vi "滤波参数.vi"(7 "滤波次数":u32=5, 11 "x":dbl format="%0.2f") -> (3 "mode":dbl caption="众数" format="%0.2f")   [LabVIEW 2016, in "斯坦道多参数.lvlib"]
uses:
  <vilib>/Analysis/baseanly.llb/Mean (DBL).vi
  <vilib>/Analysis/NI_AALBase.lvlib
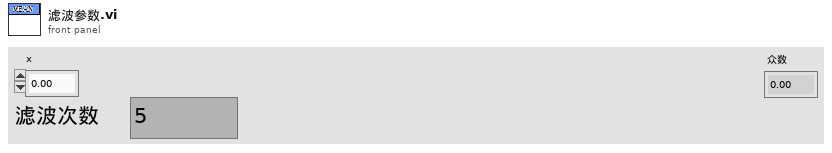
[diagram p1: front panel]
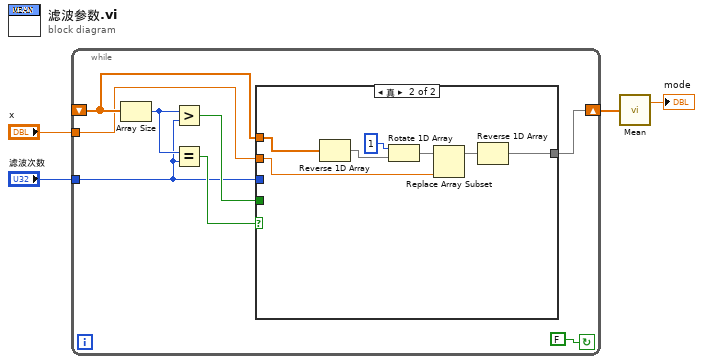
[diagram p0: block diagram]
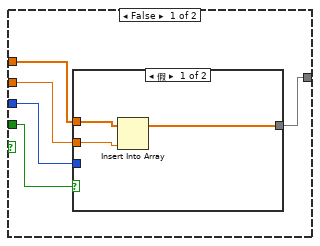
[diagram p2: hidden frame]
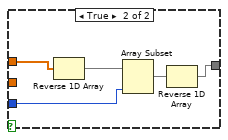
[diagram p3: hidden frame]
diagram:
  n1 = while {
    tunnel: "滤波次数" -> [w5]
    tunnel: "x" -> [w9]
    shift-right: [w8] -> w2
    shift-left: _ -> [w10]
    stop <- FALSE continue-if-true
    n2 = Array Size(array=w10) -> (size(s)=w7:i32)
    n3 = Greater?(x=w7, y=w5) -> (0:w6:bool)
    n4 = Equal?(x=w7, y=w5) -> (x = y?=w11:bool)
    n5 = case shown="真" w11 {
      tunnel: w10 -> [w17 w32]
      tunnel: w9 -> [w16 w30]
      tunnel: [w15 w26] -> w8
      tunnel: w6 -> [w14 _]
      tunnel: w5 -> [w13 _]
      frame False {
        n6 = case shown="假" w14 {
          tunnel: w17 -> [w20 w25]
          tunnel: w16 -> [w19 _]
          tunnel: [w18 w21] -> w15
          tunnel: w13 -> [_ w23]
          frame False {
            n7 = Insert Into Array(array=w20, new element=w19) -> (w18:dbl[])  [unwired: 1 in]
          }
          frame True {
            n8 = Reverse 1D Array(array=w25) -> (reversed array=w24:dbl[])
            n9 = Array Subset(array=w24, length=w23) -> (w22:dbl[])  [unwired: 1 in]
            n10 = Reverse 1D Array(array=w22) -> (reversed array=w21:dbl[])
          }
        }
      }
      frame True {
        n11 = Reverse 1D Array(array=w32) -> (reversed array=w27:dbl[])
        n12 = Rotate 1D Array(1:w27, 2:1 ("n")) -> (0:w31:dbl[])
        n13 = Replace Array Subset(array=w31, new element=w30) -> (w29:dbl[])  [unwired: 1 in]
        n14 = Reverse 1D Array(array=w29) -> (reversed array=w26:dbl[])
      }
    }
  }
  n15 = call-poly <vilib>:"Mean.vi"("X"=w2) -> ("mean"=→"mode":dbl)  [unwired: 1 out]
